vi "Bias Control.vi"(5 "error in (no error)":errorcluster, 6 "Minimum Voltage Magnitude\n(DO NOT SET TO 0)":dbl=0.1 format="%#_6p", 7 "Voltage Slew Rate (Volts/second)":dbl=1.0 min=0.0 format="%#_6p", 8 "Voltage Bias":dbl=1.0 format="%#_6p") -> (0 "error out":errorcluster)   [LabVIEW 2017]
uses:
  <userlib>/Nanonis Prog Interface/Nanonis Prog Interface.lvlib
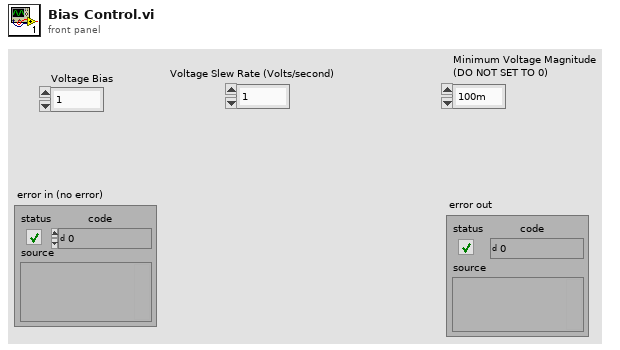
[diagram p1: front panel]
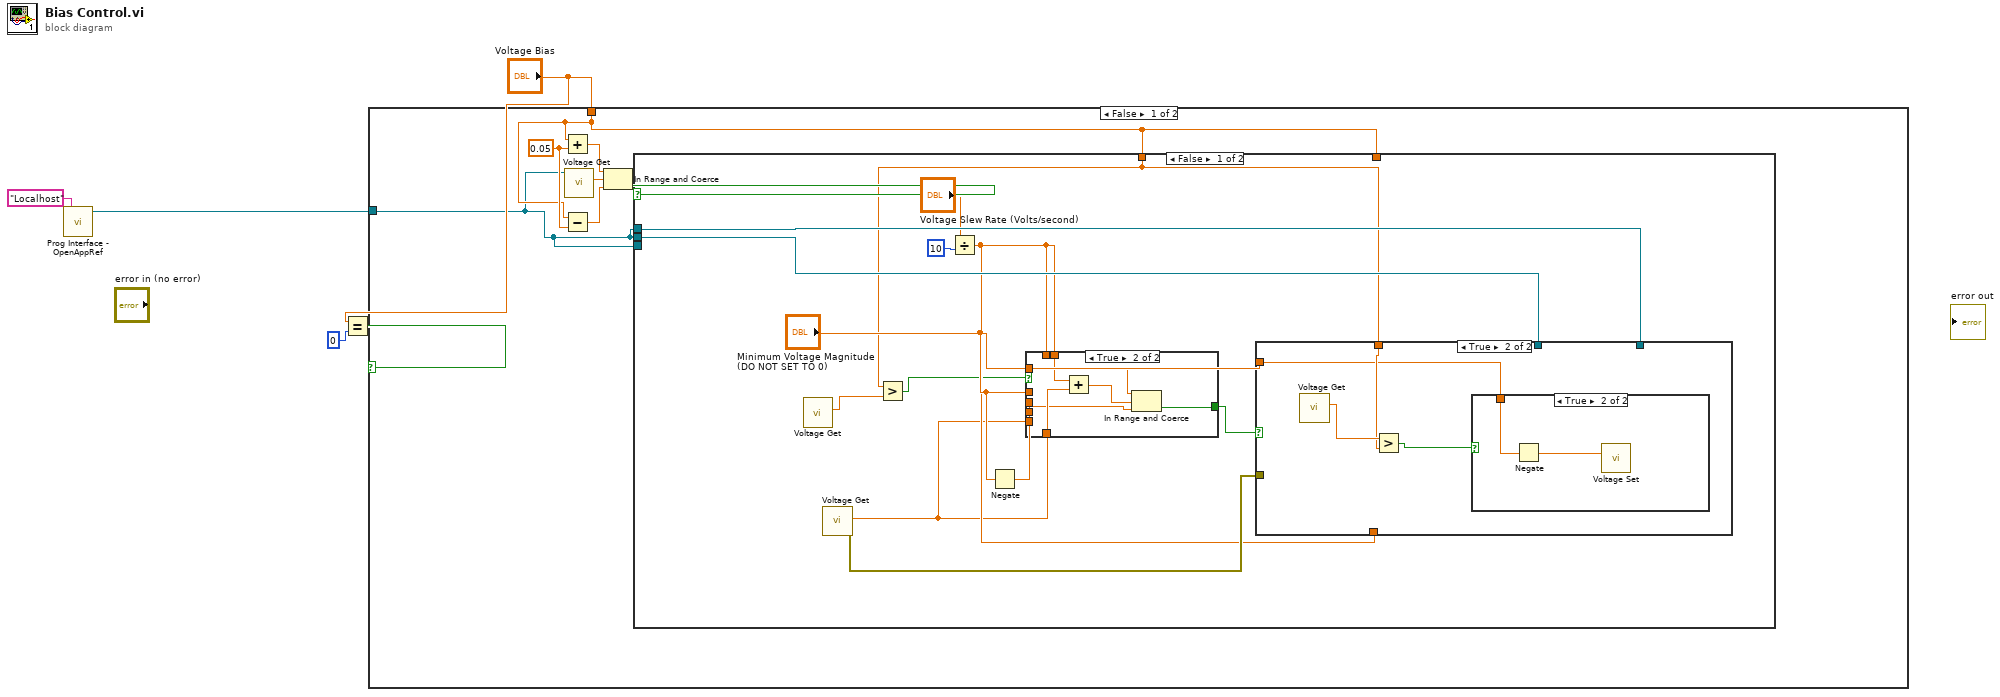
[diagram p0: block diagram]
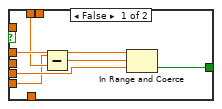
[diagram p2: hidden frame]
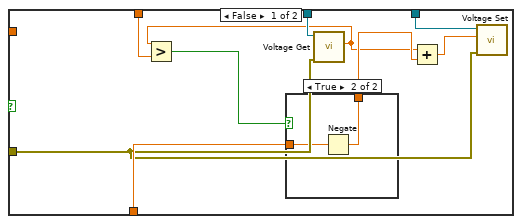
[diagram p3: hidden frame]
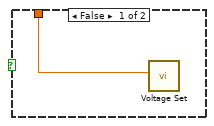
[diagram p5: hidden frame]
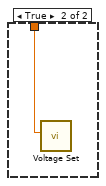
[diagram p6: hidden frame]
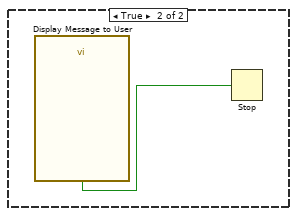
[diagram p7: hidden frame]
diagram:
  n1 = call <userlib>:"Prog Interface - OpenAppRef.vi"("Machine name (local machine IP)"="Localhost") -> ("Application reference"=w4:refnum<vi>)  [unwired: 5 in, 1 out]
  n2 = Equal?(x="Voltage Bias", y=0) -> (x = y?=w1:bool)
  n3 = case shown="False" w1 {
    tunnel: w4 -> [w6 _]
    tunnel: "Voltage Bias" -> [w7 _]
    frame False {
      w9 = 0.05
      n4 = Add(x=w7, y=w9) -> (x+y=w11:dbl)
      n5 = Subtract(x=w7, y=w9) -> (x-y=w12:dbl)
      n6 = call <userlib>:"Voltage Get.vi"("Application ref in"=w6) -> ("Bias (V)"=w10:sgl)  [unwired: 8 in, 2 out]
      n7 = In Range and Coerce(upper limit=w11, x=w10, lower limit=w12) -> (In Range?=w8:bool)  [unwired: 1 out]
      n8 = case shown="False" w8 {
        tunnel: w6 -> [_ _]
        tunnel: w7 -> [_ w57]
        tunnel: w7 -> [w15 _]
        tunnel: w6 -> [w23 _]
        tunnel: w6 -> [w22 _]
        frame False {
          n9 = call <userlib>:"Voltage Get.vi"() -> ("Bias (V)"=w14:sgl)  [unwired: 9 in, 2 out]
          n10 = call <userlib>:"Voltage Get.vi"() -> ("error out"=w24:errorcluster, "Bias (V)"=w17:sgl)  [unwired: 9 in, 1 out]
          n11 = Greater?(x=w15, y=w14) -> (0:w13:bool)
          n12 = Divide(x="Voltage Slew Rate (Volts/second)", y=10) -> (x/y=w18:dbl)
          n13 = Negate(x="Minimum Voltage Magnitude\n(DO NOT SET TO 0)") -> (-x=w20:dbl)
          n14 = case shown="True" w13 {
            tunnel: w18 -> [_ w37]
            tunnel: w17 -> [_ w36]
            tunnel: w20 -> [_ w35]
            tunnel: "Minimum Voltage Magnitude\n(DO NOT SET TO 0)" -> [_ w33]
            tunnel: w20 -> [w31 _]
            tunnel: "Minimum Voltage Magnitude\n(DO NOT SET TO 0)" -> [w30 _]
            tunnel: w18 -> [w29 _]
            tunnel: w17 -> [w28 _]
            tunnel: [w26 w32] -> w16
            frame False {
              n15 = Subtract(x=w28, y=w29) -> (x-y=w27:dbl)
              n16 = In Range and Coerce(upper limit=w30, x=w27, lower limit=w31) -> (In Range?=w26:bool)  [unwired: 1 out]
            }
            frame True {
              n17 = Add(x=w37, y=w36) -> (x+y=w34:dbl)
              n18 = In Range and Coerce(upper limit=w33, x=w34, lower limit=w35) -> (In Range?=w32:bool)  [unwired: 1 out]
            }
          }
          n19 = case shown="True" w16 {
            tunnel: w15 -> [w46 w52]
            tunnel: "Minimum Voltage Magnitude\n(DO NOT SET TO 0)" -> [_ w50]
            tunnel: w18 -> [w44 _]
            tunnel: w24 -> [w40 _]
            tunnel: w23 -> [w41 _]
            tunnel: w22 -> [w39 _]
            frame False {
              n20 = call <userlib>:"Voltage Get.vi"("error in (no error)"=w40, "Application ref in"=w41) -> ("Bias (V)"=w38:sgl)  [unwired: 7 in, 2 out]
              n21 = Greater?(x=w38, y=w46) -> (0:w45:bool)
              n22 = case shown="True" w45 {
                tunnel: w44 -> [w47 w49]
                tunnel: [w47 w48] -> w42
                frame False {
                }
                frame True {
                  n23 = Negate(x=w49) -> (-x=w48:dbl)
                }
              }
              n24 = Add(x=w38, y=w42) -> (x+y=w43:dbl)
              n25 = call <userlib>:"Voltage Set.vi"("Error in (no error)"=w40, "Bias (V)"=w43, "Application ref in"=w39) -> ()  [unwired: 7 in, 2 out]
            }
            frame True {
              n26 = call <userlib>:"Voltage Get.vi"() -> ("Bias (V)"=w53:sgl)  [unwired: 9 in, 2 out]
              n27 = Greater?(x=w53, y=w52) -> (0:w51:bool)
              n28 = case shown="True" w51 {
                tunnel: w50 -> [w54 w56]
                frame False {
                  n29 = call <userlib>:"Voltage Set.vi"("Bias (V)"=w54) -> ()  [unwired: 9 in, 2 out]
                }
                frame True {
                  n30 = Negate(x=w56) -> (-x=w55:dbl)
                  n31 = call <userlib>:"Voltage Set.vi"("Bias (V)"=w55) -> ()  [unwired: 9 in, 2 out]
                }
              }
            }
          }
        }
        frame True {
          n32 = call <userlib>:"Voltage Set.vi"("Bias (V)"=w57) -> ()  [unwired: 9 in, 2 out]
        }
      }
    }
    frame True {
      n33 = call "Display Message to User"() -> ("OK"=w58:bool)  [unwired: 10 in, 1 out]
      n34 = Stop(stop? (T)=w58) -> ()
    }
  }
